vi "Encoders Based Driving.vi"(0 "Distance":dbl) -> (1 "Encoder Bigger Than Distance":bool, 2 "Encoder Value":dbl)   [LabVIEW 2018]
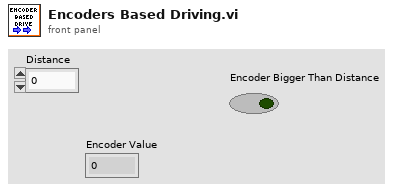
[diagram p1: front panel]
types:
  T1 = typedef "WPI_EncoderDevRef.ctl" = cluster{"DevStatus":errorcluster, "EncoderIndex":T2, "CounterIndex":T3, "DistancePerCount":dbl, "Decoding Type":T4}
  T2 = typedef "FPGA_EncoderIdx.ctl" = enum8{"Enc 0", "Enc 1", "Enc 2", "Enc 3", "Enc 4", "Enc 5", "Enc 6", "Enc 7", "Invalid"}
  T3 = typedef "FPGA_CounterCtrSystemIndex.ctl" = enum8{"Ctr 0", "Ctr 1", "Ctr 2", "Ctr 3", "Ctr 4", "Ctr 5", "Ctr 6", "Ctr 7", "Invalid"}
  T4 = typedef "WPI_EncoderType.ctl" = enum16{"1x", "2x", "4x"}
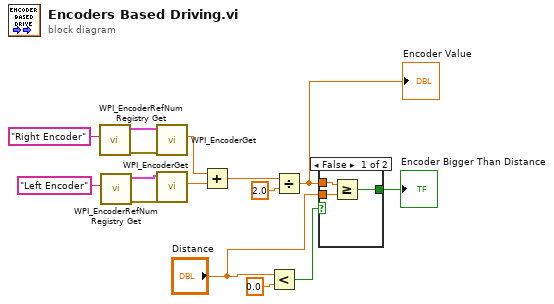
[diagram p0: block diagram]
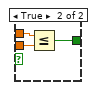
[diagram p2: hidden frame]
diagram:
  n1 = call <vilib>:"WPI_EncoderRefNum Registry Get.vi"("refnum name"="Right Encoder") -> ("error out"=w7:errorcluster, "EncoderDevRef"=w6:T1)  [unwired: 9 in]
  n2 = call <vilib>:"WPI_EncoderRefNum Registry Get.vi"("refnum name"="Left Encoder") -> ("error out"=w2:errorcluster, "EncoderDevRef"=w3:T1)  [unwired: 9 in]
  n3 = call <vilib>:"WPI_EncoderGet.vi"("error in (no error)"=w7, "EncoderDevRef"=w6) -> ("Distance"=w15:dbl)  [unwired: 4 in, 5 out]
  n4 = call <vilib>:"WPI_EncoderGet.vi"("error in (no error)"=w2, "EncoderDevRef"=w3) -> ("Distance"=w14:dbl)  [unwired: 4 in, 5 out]
  n5 = Add(x=w15, y=w14) -> (x+y=w13:dbl)
  n6 = Less?(x="Distance", y=0.0) -> (x < y?=w9:bool)
  n7 = Divide(x=w13, y=2.0) -> (x/y=w1:dbl)
  "Encoder Value" <- w1
  n8 = case shown="False" w9 {
    tunnel: "Distance" -> [w17 w21]
    tunnel: w1 -> [w18 w20]
    tunnel: [w16 w19] -> w8
    frame False {
      n9 = Greater Or Equal?(x=w18, y=w17) -> (x >= y?=w16:bool)
    }
    frame True {
      n10 = Less Or Equal?(x=w20, y=w21) -> (x <= y?=w19:bool)
    }
  }
  "Encoder Bigger Than Distance" <- w8
